vi "Close SV.vi"(8 "error in (no error)":errorcluster, 10 "Process Name":string="Flow Module 1", 11 "State Cluster in":T17={"PRM Config"={"GUID"="PID1-Mettler Toledo Scale 1", "Drop Coords"={"Horizontal"=0, "Vertical"=0}, "Process Name"="PID1-Setpoint", "Settings"={"Cycle Period"=500.0, "PID 2 Parameters"={"Input Device"=enum."Default", "Output Device"=enum."Default", "Setpoint"=0.0, "PID gains"={"proportional gain (Kc)"=1.0, "integral time (Ti, min)"=0.01, "derivative time (Td, min)"=0.0}}, "Manual Entry"=0.0, "Auto?"=TRUE, "output range"={"output high"=100.0, "output low"=0.0}, {"Input Channel "=0}}, "Settings Load Count"=0}} {"PRM Config"."Settings"."output range"."output low" min=0.0 max=100.0 format="%.2f"; "PRM Config"."Settings"."output range"."output high" format="%.2f"; "PRM Config"."Settings"."PID 2 Parameters"."PID gains"."derivative time (Td, min)" format="%.3f"; "PRM Config"."Settings"."PID 2 Parameters"."PID gains"."integral time (Ti, min)" format="%.3f"; "PRM Config"."Settings"."PID 2 Parameters"."PID gains"."proportional gain (Kc)" format="%.3f"}) -> (0 "error out":errorcluster, 3 "State Cluster out":T1={"Shared Variables"={"PID 1 Process Variable"="PID1-Mettler Toledo Scale 1", "PID 1 Output"="PID1-Mettler Toledo Scale 1", "PID 1 Setpoint"="PID1-Setpoint", "PID 1 Setpoint SV refnum"="ni.var.psp://localhost/Flow Module 1/PID1-Setpoint", "PID 1 Process Variable SV refnum"="ni.var.psp://localhost/Flow Module 1/PID1-Setpoint", "PID 1 Output SV refnum"="ni.var.psp://localhost/Flow Module 1/PID1-Setpoint"}, "Pressure Regulator Module Config"={"GUID"="", "Drop Coords"={"Horizontal"=0, "Vertical"=0}, "Process Name"="", "Settings"={"Cycle Period"=500.0, "Ismatech"={"VISA resource name"="", "Simulated?"=TRUE, "Pump Number"=1.0, "Reverse?"=FALSE}, "Masterflex"={"VISA resource name"="", "Simulated?"=TRUE, "Pump Number"=1.0, "Reverse?"=FALSE}, "Mettler"={"VISA resource name"="", "Simulated?"=FALSE}, "Bronkhorst M13 Flow Meter"={"VISA resource name"="", "Simulated?"=TRUE}, "PID 2 Parameters"={"Input Device"=enum."Default", "Output Device"=enum."Default", "Setpoint"=0.0, "PID gains"={"proportional gain (Kc)"=1.0, "integral time (Ti, min)"=0.01, "derivative time (Td, min)"=0.0}}, "Manual Entry"=0.0, "Auto?"=TRUE, "output range"={"output high"=100.0, "output low"=0.0}, "Bronkhorst M14"={"VISA resource name"="", "Simulated?"=FALSE}, "Tacmina Settings"={"Analog DAQ Task"="", "Digital DAQ Task"=""}, "KNF SIMDOS Settings"={"VISA resource name"="", "Simulated?"=TRUE}, "ASIA Pump C"={"ASIA Pump #"=0, "channel"=0, "Simulated"=FALSE}, "VICI M50 Settings"={"VISA resource name"="", "Simulated?"=TRUE, "Pump Letter"="", "Reverse?"=FALSE}}, "Settings Load Count"=0}} {"Pressure Regulator Module Config"."Settings"."ASIA Pump C"."channel" min=0 max=1 step=1; "Pressure Regulator Module Config"."Settings"."output range"."output low" min=0.0 max=100.0 format="%.2f"; "Pressure Regulator Module Config"."Settings"."output range"."output high" format="%.2f"; "Pressure Regulator Module Config"."Settings"."PID 2 Parameters"."PID gains"."derivative time (Td, min)" format="%.3f"; "Pressure Regulator Module Config"."Settings"."PID 2 Parameters"."PID gains"."integral time (Ti, min)" format="%.3f"; "Pressure Regulator Module Config"."Settings"."PID 2 Parameters"."PID gains"."proportional gain (Kc)" format="%.3f"; "Pressure Regulator Module Config"."Settings"."Masterflex"."Pump Number" min=1.0 max=20.0 step=1.0; "Pressure Regulator Module Config"."Settings"."Ismatech"."Pump Number" min=1.0 max=20.0 step=1.0})   [LabVIEW 2018, in "4-20mA Module.lvlib"]
uses:
  4-20mA Module.lvlib
  Shared Variables/Dynamic Shared Variables.lvlib
  Controls/Pressure Regulator Module Shared Variable Cluster.ctl
  Controls/4-20mA Module Settings Cluster.ctl
  Controls/4-20mA Module State Cluster.ctl
  Ismatec ISM 831C/Controls/Ismatech Settings Cluster.ctl
  Ismatec ISM 831C/Ismatec ISM 831C.lvlib
  Masterflex 7550-30/Controls/Settings Cluster.ctl
  Masterflex 7550-30/Masterflex 7550-30.lvlib
  Mettler Toledo/Controls/Settings Cluster.ctl
  Mettler Toledo/Mettler Toledo.lvlib
  Bronkhorst M13 Flow Meter/Settings Cluster.ctl
  Bronkhorst M13 Flow Meter/Bronkhorst M13 Flow Meter.lvlib
  Measure Instrument/PID Input Enum.ctl
  Measure Instrument/PID 2 Output Enum.ctl
  Measure Instrument/PID 2 Parameters Cluster.ctl
  <vilib>/Utility/miscctls.llb/LVPoint32TypeDef.ctl
  Controls/4-20mA Module Config Cluster.ctl
  Tacmina QI/Tacmina QI DAQ Setting.ctl
  Tacmina QI/Tacmina QI.lvlib
  KNF Pump/Settings Cluster plus SIMDOS.ctl
  KNF Pump/KNF SIMDOS.lvlib
  ASIA Pump/Pump Settings.ctl
  ASIA Pump.lvlib
  VICI M50 Party Mode/Settings Cluster.ctl
  VICI M50 Party Mode/VICI M6 M50 Party Mode.lvlib
  Pressure Transmitter/Pressure Transmitter Device Settings.ctl
  Pressure Transmitter/Pressure Transmitter Library.lvlib
panel:
  # "Output Instruments"
  # "Input Instruments"
  # "Instrument Settings"
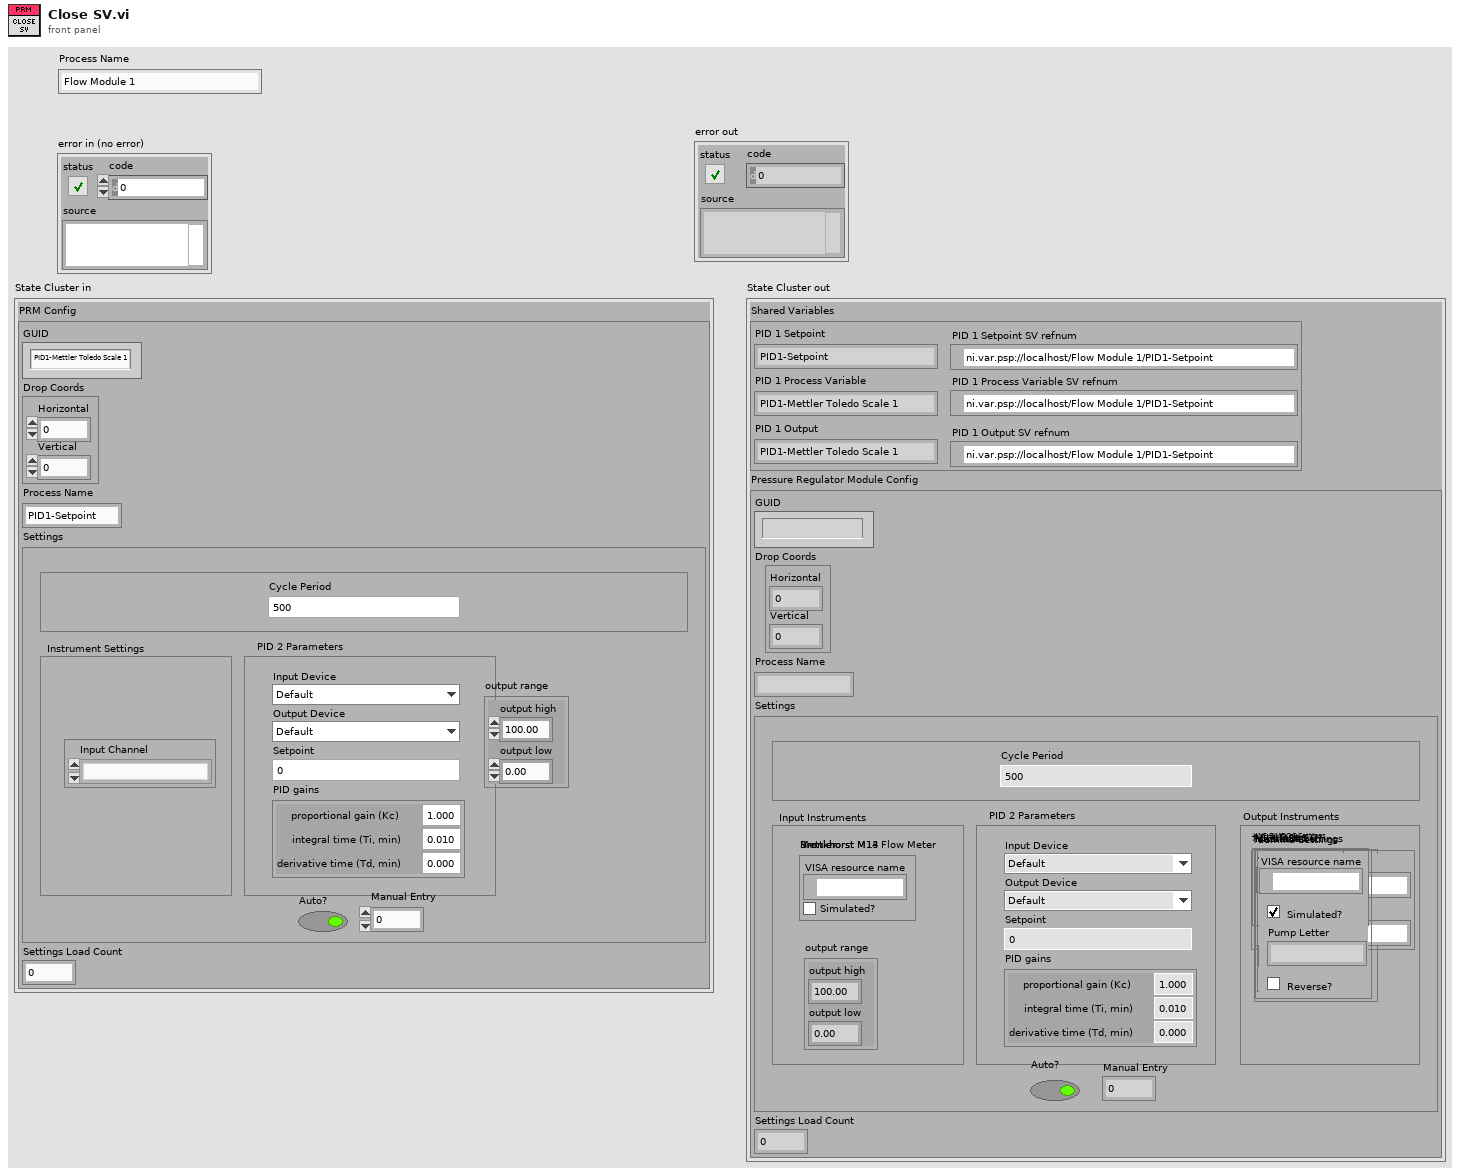
[diagram p1: front panel]
types:
  T1 = typedef "4-20mA Module.lvlib/4-20mA Module State Cluster.ctl" = cluster{"Shared Variables":T2, "Pressure Regulator Module Config":T3}
  T2 = typedef "Pressure Regulator Module Shared Variable Cluster.ctl" = cluster{"PID 1 Process Variable":string, "PID 1 Output":string, "PID 1 Setpoint":string, "PID 1 Setpoint SV refnum":refnum<k21>, "PID 1 Process Variable SV refnum":refnum<k21>, "PID 1 Output SV refnum":refnum<k21>}
  T3 = typedef "4-20mA Module.lvlib/4-20mA Module Config Cluster.ctl" = cluster{"GUID":string, "Drop Coords":T4, "Process Name":string, "Settings":T5, "Settings Load Count":i32}
  T4 = typedef "LVPoint32TypeDef.ctl" = cluster{"Horizontal":i32, "Vertical":i32}
  T5 = typedef "4-20mA Module.lvlib/4-20mA Module Settings Cluster.ctl" = cluster{"Cycle Period":dbl, "Ismatech":T6, "Masterflex":T7, "Mettler":T8, "Bronkhorst M13 Flow Meter":T9, "PID 2 Parameters":T10, "Manual Entry":dbl, "Auto?":bool, "output range":cluster{"output high":dbl, "output low":dbl}, "Bronkhorst M14":T8, "Tacmina Settings":T13, "KNF SIMDOS Settings":T14, "ASIA Pump C":T15, "VICI M50 Settings":T16}
  T6 = typedef "Ismatec ISM 831C.lvlib/Ismatech Settings Cluster.ctl" = cluster{"VISA resource name":refnum<visa-resource-name>, "Simulated?":bool, "Pump Number":dbl, "Reverse?":bool}
  T7 = typedef "Masterflex 7550-30.lvlib/Settings Cluster.ctl" = cluster{"VISA resource name":refnum<visa-resource-name>, "Simulated?":bool, "Pump Number":dbl, "Reverse?":bool}
  T8 = typedef "Mettler Toledo.lvlib/Settings Cluster.ctl" = cluster{"VISA resource name":refnum<visa-resource-name>, "Simulated?":bool}
  T9 = typedef "Bronkhorst M13 Flow Meter.lvlib/Settings Cluster.ctl" = cluster{"VISA resource name":refnum<visa-resource-name>, "Simulated?":bool}
  T10 = typedef "PID 2 Parameters Cluster.ctl" = cluster{"Input Device":T11, "Output Device":T12, "Setpoint":dbl, "PID gains":cluster{"proportional gain (Kc)":dbl, "integral time (Ti, min)":dbl, "derivative time (Td, min)":dbl}}
  T11 = typedef "PID Input Enum.ctl" = enum16{"Default", "Bronkhorst M13", "Bronkhorst M14", "Scale Rate of Change"}
  T12 = typedef "PID 2 Output Enum.ctl" = enum16{"Default", "Ismatec ISM 831C", "Masterflex 7550-30", "VICI M50", "Tacmina QI", "KNF SIMDOS", "ASIA Type C", "FLOM UI-22-11", "SSI PR"}
  T13 = typedef "Tacmina QI.lvlib/Tacmina QI DAQ Setting.ctl" = cluster{"Analog DAQ Task":refnum<k21>, "Digital DAQ Task":refnum<k21>}
  T14 = typedef "KNF SIMDOS.lvlib/Settings Cluster plus SIMDOS.ctl" = cluster{"VISA resource name":refnum<visa-resource-name>, "Simulated?":bool}
  T15 = typedef "ASIA Pump.lvlib/Pump Settings.ctl" = cluster{"ASIA Pump #":i32, "channel":i32, "Simulated":bool}
  T16 = typedef "VICI M6 M50 Party Mode.lvlib/Settings Cluster.ctl" = cluster{"VISA resource name":refnum<visa-resource-name>, "Simulated?":bool, "Pump Letter":string, "Reverse?":bool}
  T17 = typedef "4-20mA Module.lvlib/4-20mA Module State Cluster.ctl" = cluster{"PRM Config":T18}
  T18 = typedef "4-20mA Module.lvlib/4-20mA Module Config Cluster.ctl" = cluster{"GUID":string, "Drop Coords":T4, "Process Name":string, "Settings":T19, "Settings Load Count":i32}
  T19 = typedef "4-20mA Module.lvlib/4-20mA Module Settings Cluster.ctl" = cluster{"Cycle Period":dbl, "PID 2 Parameters":cluster{"Input Device":enum16{"Default", "4-20mA"}, "Output Device":enum16{"Default", "4-20mA"}, "Setpoint":dbl, "PID gains":cluster{"proportional gain (Kc)":dbl, "integral time (Ti, min)":dbl, "derivative time (Td, min)":dbl}}, "Manual Entry":dbl, "Auto?":bool, "output range":cluster{"output high":dbl, "output low":dbl}, T20}
  T20 = typedef "Pressure Transmitter Library.lvlib/Pressure Transmitter Device Settings.ctl" = cluster{"Input Channel ":u16}
  T21 = typedef "Pressure Regulator Module.lvlib/Pressure Regulator Module Shared Variable Cluster.ctl" = cluster{"PID 1 Process Variable":string, "PID 1 Output":string, "PID 1 Setpoint":string, "PID 1 Setpoint SV refnum":refnum<k21>, "PID 1 Process Variable SV refnum":refnum<k21>, "PID 1 Output SV refnum":refnum<k21>}
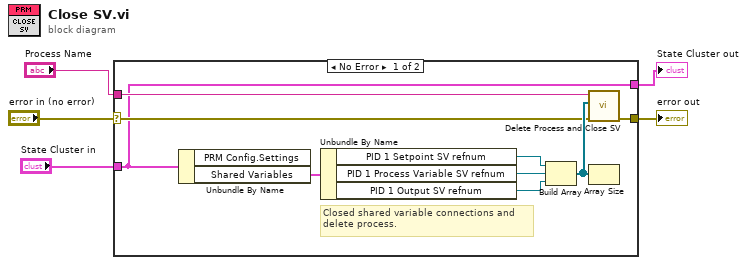
[diagram p0: block diagram]
diagram:
  n1 = case shown="No Error" "error in (no error)" {
    selector: "error in (no error)" -> [w8 w16]
    tunnel: "Process Name" -> [w13 _]
    tunnel: [w7 w16] -> w3
    tunnel: "State Cluster in" -> [w6 w15]
    tunnel: [w6 w15] -> w1
    frame No Error {
      # "Closed shared variable connections and\ndelete process."
      n2 = Unbundle By Name(w6) -> ("Shared Variables"=w14:T21)  [unwired: 1 out]
      n3 = Unbundle By Name(w14) -> ("PID 1 Setpoint SV refnum"=w12:refnum<k21>, "PID 1 Process Variable SV refnum"=w11:refnum<k21>, "PID 1 Output SV refnum"=w10:refnum<k21>)
      n4 = Build Array(w12, w11, w10) -> (w9:refnum<k21>[])
      n5 = call "Delete Process and Close SV.vi"("error in (no error)"=w8, "Array"=w9, "process name"=w13) -> ("error out"=w7:errorcluster)  [unwired: 8 in]
      n6 = Array Size(array=w9) -> ()  [unwired: 1 out]
    }
    frame Error {
    }
  }
  "error out" <- w3
  "State Cluster out" <- w1
